vi "Exp no 9 Fibonacci Series.vi"() -> ()   [LabVIEW 2010]
panel:
  out "Fibonacci Series":i32[](array[numeric])
  in  "Input N":i32
  # "FIBONACCI SERIES"
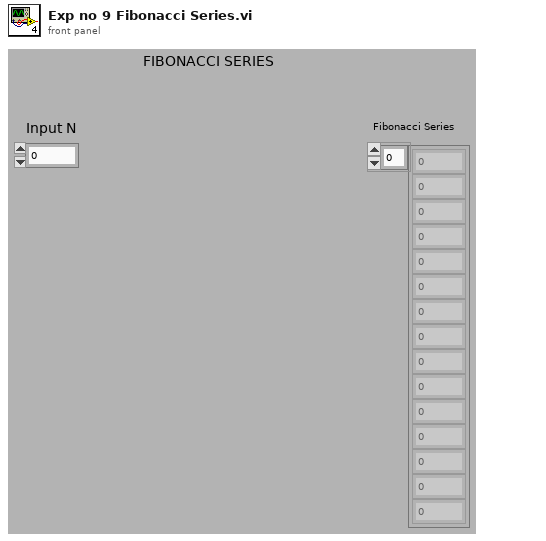
[diagram p1: front panel]
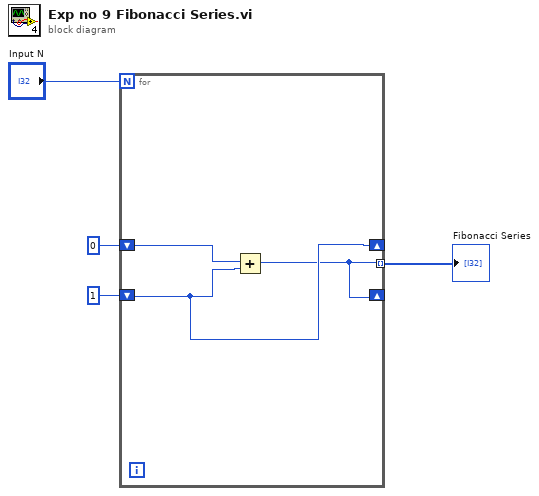
[diagram p0: block diagram]
diagram:
  n1 = for {
    N: "Input N" -> [_]
    tunnel: [w5] -> w2 mode=indexing
    shift-right: [w6] -> _
    shift-left: 0 ("x+y") -> [w7]
    shift-right: [w5] -> _
    shift-left: 1 ("y") -> [w6]
    n2 = Add(x=w7, y=w6) -> (x+y=w5:i32)
  }
  "Fibonacci Series" <- w2
